vi "Post-Build Action_Make copy for LV2015.vi"(5 "Files Generated by Build":path[](array[path]), 6 "Top Level/Always Included VIs":path[](array[path]), 7 "Destination Path":path, 8 "error in (no error)":errorcluster, 9 "Target Name":string, 10 "Build Specification Name":string, 11 "Project Path":path) -> (0 "error out":errorcluster)   [LabVIEW 2023]
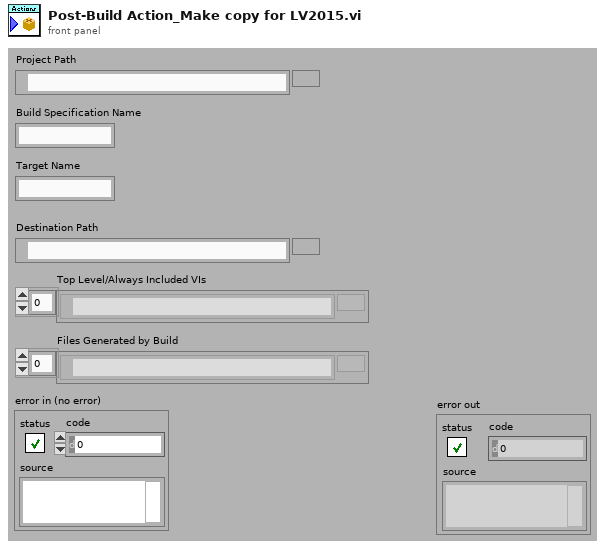
[diagram p1: front panel]
types:
  T1 = enum16{"Stop on First Error and report", "Continue on Error and Report", "Clear all Errors"}
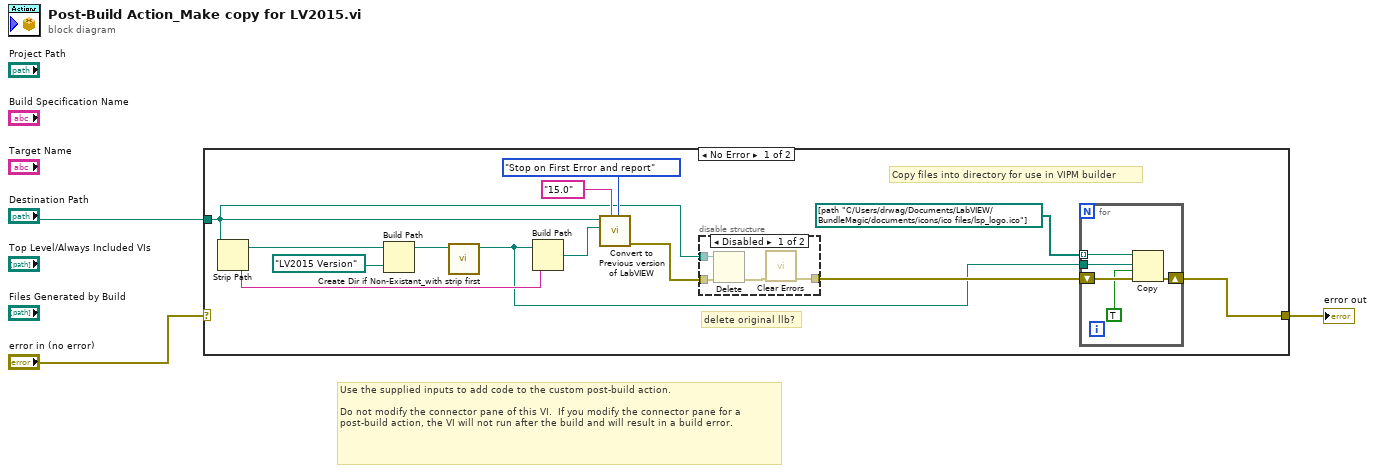
[diagram p0: block diagram]
diagram:
  # "Use the supplied inputs to add code to the custom post-build action.\n\nDo not modify the connector pane of this VI.  If you modify the connector pane for a post-build action, the VI will not run after the build and will result in a build error."
  n1 = case shown="No Error" "error in (no error)" {
    selector: "error in (no error)" -> [_ w27]
    tunnel: "Destination Path" -> [w7 _]
    tunnel: [w8 w27] -> w1
    frame No Error {
      # "delete original llb?"
      # "Copy files into directory for use in VIPM builder"
      n2 = Strip Path(path=w7) -> (stripped path=w11:path, name=w14:string)
      n3 = Build Path(base path=w11, name or relative path=path "LV2015 Version") -> (appended path=w5:path)
      n4 = call "Create Dir if Non-Existant_with strip first.vi"("Directory Path"=w5) -> ("dup Directory Path"=w4:path)  [unwired: 8 in, 2 out]
      n5 = Build Path(base path=w4, name or relative path=w14) -> (appended path=w10:path)
      n6 = call "Convert to Previous version of LabVIEW.vi"("Error Handling"=T1."Stop on First Error and report", "Previous Version"="15.0", "Destination for down converted files."=w10, "Folder of LabVIEW files"=w7) -> ("error out"=w12:errorcluster)  [unwired: 6 in, 1 out]
      n7 = disable-structure shown="Disabled" {
        disable-tunnel: w12 -> [w19 w21]
        disable-tunnel: w7 -> [w18 _]
        disable-tunnel: [w17 w21] -> w6
        frame Disabled {
          n8 = Delete(path (use dialog)=w18, error in=w19) -> (error out=w20:errorcluster)  [unwired: 3 in, 2 out]
          n9 = call <vilib>:"Clear Errors.vi"("error in (no error)"=w20) -> ("error out"=w17:errorcluster)  [unwired: 5 in, 1 out]
        }
        frame Enabled {
        }
      }
      n10 = for {
        shift-right: [w25] -> w8
        shift-left: w6 -> [w26]
        tunnel: path[] [path "C:/Users/drwag/Documents/LabVIEW/BundleMagic/documents/icons/ico files/lsp_logo.ico"] ("name or relative path") -> [w24] mode=indexing
        tunnel: w4 -> [w23]
        n11 = Copy(8:w26, 9:TRUE ("overwrite (F)"), 10:w23, 11:w24) -> (0:w25:errorcluster)  [unwired: 1 in, 2 out]
      }
    }
    frame Error {
    }
  }
  "error out" <- w1
